vi "controlFrequenzy.vi"(7 "Set":bool, 8 "error in":errorcluster, 9 "Frequenzy [Hz] in":dbl, 10 "axis in":u8, 11 "connection ID":refnum<k5>) -> (0 "error out":errorcluster, 1 "Frequenzy [Hz] out":dbl, 2 "axis out":u8, 3 "connection ID":refnum<k5>)   [LabVIEW 2019]
panel:
  in  "Set Command":string="com.attocube.amc.control.setControlFrequency"
  in  "Get Command":string="com.attocube.amc.control.getControlFrequency"
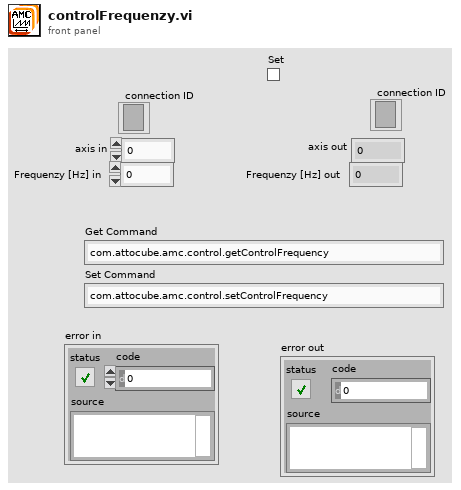
[diagram p1: front panel]
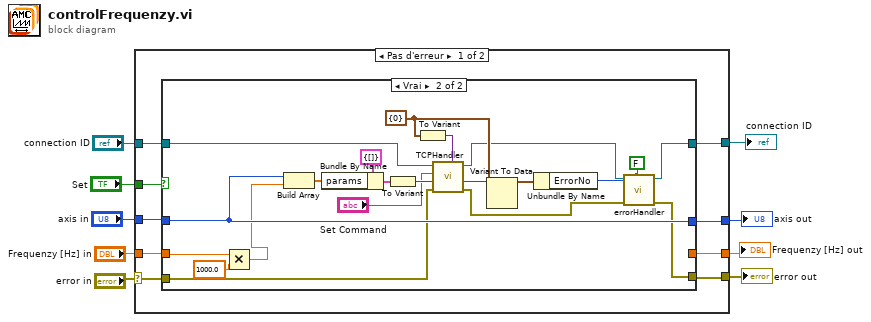
[diagram p0: block diagram]
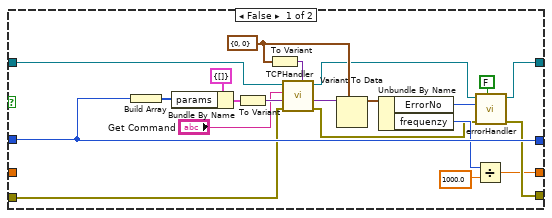
[diagram p2: hidden frame]
diagram:
  n1 = case shown="Pas d'erreur" "error in" {
    selector: "error in" -> [w14 w64]
    tunnel: "axis in" -> [w16 w62]
    tunnel: [w10 w64] -> w8
    tunnel: [w12 w62] -> w7
    tunnel: "Frequenzy [Hz] in" -> [w15 w63]
    tunnel: [w11 w63] -> w5
    tunnel: "Set" -> [w17 _]
    tunnel: [w13 w61] -> w3
    tunnel: "connection ID" -> [w18 w61]
    frame No Error {
      n2 = case shown="Vrai" w17 {
        tunnel: [w22 w43] -> w13
        tunnel: w18 -> [w29 w55]
        tunnel: w16 -> [w31 w53]
        tunnel: [w31 w53] -> w12
        tunnel: [w30 w50] -> w10
        tunnel: [w24 _] -> w11
        tunnel: w15 -> [_ w45]
        tunnel: w14 -> [w20 w41]
        frame False {
          w27 = cluster{"ErrorNo":i16, "frequenzy":i64} {"ErrorNo"=0, "frequenzy"=0} ("input cluster")
          n3 = Build Array(w31) -> (w35:u8[])
          n4 = Bundle By Name(cluster=cluster{"params":i16[]} {"params"=[]} ("input cluster"), "params"=w35) -> (w36:cluster{"params":i16[]})
          n5 = To Variant(anything=w36) -> (Variant=w37:variant)
          n6 = To Variant(anything=w27) -> (Variant=w28:variant)
          n7 = call <userlib>:"TCPHandler.vi"("result Types"=w28, "error in (no error)"=w20, "params"=w37, "method"="Get Command", "connection ID"=w29) -> ("error out"=w19:errorcluster, "result"=w33:variant, "connection ID"=w23:refnum<k5>)  [unwired: 3 in, 1 out]
          n8 = Variant To Data(type=w27, Variant=w33) -> (data=w38:cluster{"ErrorNo":i16, "frequenzy":i64})  [unwired: 1 in, 1 out]
          n9 = Unbundle By Name(w38) -> ("ErrorNo"=w39:i16, "frequenzy"=w25:i64)
          n10 = Divide(x=w25, y=1000.0) -> (x/y=w24:dbl)
          n11 = call <userlib>:"errorHandler.vi"("show popup"=FALSE, "error in"=w19, "error number"=w39, "connection ID"=w23) -> ("error out"=w30:errorcluster, "connection ID"=w22:refnum<k5>)  [unwired: 6 in]
        }
        frame True {
          w48 = cluster{"ErrorNo":i16} {"ErrorNo"=0} ("input cluster")
          n12 = Multiply(x=w45, y=1000.0) -> (x*y=w46:dbl)
          n13 = Build Array(w53, w46) -> (w57:dbl[])
          n14 = Bundle By Name(cluster=cluster{"params":i64[]} {"params"=[]} ("input cluster"), "params"=w57) -> (w56:cluster{"params":i64[]})
          n15 = To Variant(anything=w56) -> (Variant=w54:variant)
          n16 = To Variant(anything=w48) -> (Variant=w49:variant)
          n17 = call <userlib>:"TCPHandler.vi"("result Types"=w49, "error in (no error)"=w41, "params"=w54, "method"="Set Command", "connection ID"=w55) -> ("error out"=w40:errorcluster, "result"=w59:variant, "connection ID"=w44:refnum<k5>)  [unwired: 3 in, 1 out]
          n18 = Variant To Data(type=w48, Variant=w59) -> (data=w52:cluster{"ErrorNo":i16})  [unwired: 1 in, 1 out]
          n19 = Unbundle By Name(w52) -> ("ErrorNo"=w51:i16)
          n20 = call <userlib>:"errorHandler.vi"("show popup"=FALSE, "error in"=w40, "error number"=w51, "connection ID"=w44) -> ("error out"=w50:errorcluster, "connection ID"=w43:refnum<k5>)  [unwired: 6 in]
        }
      }
    }
    frame Error {
    }
  }
  "error out" <- w8
  "axis out" <- w7
  "Frequenzy [Hz] out" <- w5
  "connection ID" <- w3
